vi "CRYGet DataView Arrary Idx.vi"(11 "DataView Idx In":i32) -> (3 "DataView Arrary Idx out":i32)   [LabVIEW 2013]
uses:
  CRYNew View Global.vi
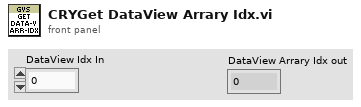
[diagram p1: front panel]
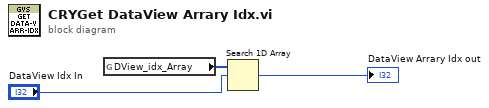
[diagram p0: block diagram]
diagram:
  n1 = global read "CRYNew View Global.vi" "DView_idx_Array"() -> (w3:i32[])
  n2 = Search 1D Array(1D array=w3, element="DataView Idx In") -> (index of element=→"DataView Arrary Idx out":i32)  [unwired: 1 in]
